vi "Write Dependencies' Unique Names.vi"(8 "error in (no error)":errorcluster, 10 "Dependencies' Unique Names":string[](array[string]), 11 "Export in":refnum<class "Export.lvclass">) -> (0 "error out":errorcluster, 3 "Export out":refnum<class "Export.lvclass">)   [LabVIEW 2017, in "CL_G3_VIComponentBuilder.lvlib" / "Export.lvclass"]
uses:
  Export.lvclass
  Export.lvclass/Export.ctl
  Read Export Build Specification.vi
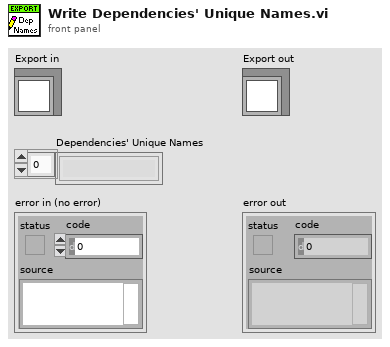
[diagram p1: front panel]
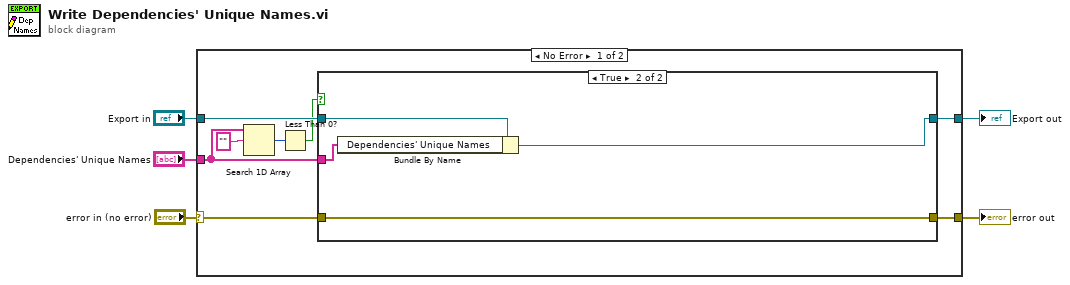
[diagram p0: block diagram]
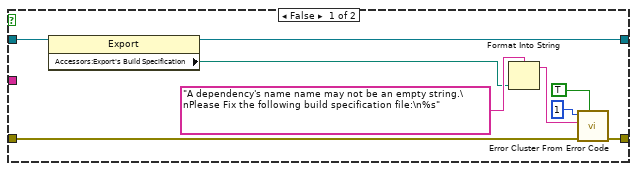
[diagram p2: hidden frame]
diagram:
  n1 = case shown="No Error" "error in (no error)" {
    selector: "error in (no error)" -> [w8 w27]
    tunnel: [w6 w27] -> w4
    tunnel: [w9 w28] -> w2
    tunnel: "Export in" -> [w10 w28]
    tunnel: "Dependencies' Unique Names" -> [w11 _]
    frame No Error {
      n2 = Search 1D Array(1D array=w11, element="") -> (index of element=w12:i32)  [unwired: 1 in]
      n3 = Less Than 0?(x=w12) -> (x < 0?=w7:bool)
      n4 = case shown="True" w7 {
        tunnel: w8 -> [w22 w26]
        tunnel: [w14 w26] -> w6
        tunnel: w10 -> [w16 w25]
        tunnel: [w17 w24] -> w9
        tunnel: w11 -> [_ w23]
        frame False {
          n5 = property class="Export"(reference=w16) -> (reference out=w17:refnum<class "Export.lvclass">, "Accessors:Export's Build Specification"=w15:path)  [unwired: 1 in, 1 out]
          n6 = Format Into String(format string="A dependency's name name may not be an empty string.\nPlease Fix the following build specification file:\n%s" ("error message (\"\")"), w15) -> (resulting string=w18:string)  [unwired: 2 in, 1 out]
          n7 = call <vilib>:"Error Cluster From Error Code.vi"("show call chain? (False)"=TRUE, "error in (no error)"=w22, "error message (\"\")"=w18, "error code (0)"=1) -> ("error out"=w14:errorcluster)  [unwired: 5 in]
        }
        frame True {
          n8 = Bundle By Name(cluster=w25, "Dependencies' Unique Names"=w23) -> (w24:refnum<class "Export.lvclass">)
        }
      }
    }
    frame Error {
    }
  }
  "error out" <- w4
  "Export out" <- w2
